vi "Main-Strech DNA-OneDirectionOnly_YCC.vi"() -> ()   [LabVIEW 2014]
uses:
  <vilib>/DAQmx/create/channels.llb/DAQmx Create Channel (AI-Voltage-Basic).vi
  <vilib>/DAQmx/configure/timing.llb/DAQmx Timing (Sample Clock).vi
  Main-Calibration/WLC fitting/SubVI/WLC-Fitting Cluster.ctl
panel:
  out "Fold QPD Signal (V) 2":dbl[](array[numeric])
  out "Fold Stage Position (um) 2":dbl[](array[numeric])
  out "Folded-Force":dbl[](array[numeric])
  out "Folded-xDNA":dbl[](array[numeric])
  out "Unfolded-Force":dbl[](array[numeric])
  out "Unfolded-xDNA":dbl[](array[numeric])
  in  "Fitting Cluster":T1={"cr (um)"=0.0, "yr (V)"=0.0, "trap height(nm)"=300.0, "bead radius(nm)"=515.0, "Length offset"=0.0, "conversion factor (V/um)"=0.0, "Force constant (pN/nm)"=0.0154, "Force offset"=500.0, "cr shift (nm)"=0.0, "yr shift (mV)"=0.0, "LaserPower (mW)"=10.0, "Cf. Calib. Array"=[0.192406, 0.0124489], "Stiffness Calib. array"=[0.004414, 0.00367]}
  out "Filtered QPD Array":dbl[][](array[numeric])
  out "Filtered Stage Array":dbl[][](array[numeric])
  out "Save to File Name Indicator":string
  out "Save to Path Indicator":path
  in  "Who's Data":enum16{"YCC", "PYW", "LCH"}(ring)
  in  "File name add to the end \n(laser power-height)":string="10mW-h300"
  in  "Save Raw Data?":bool
  out "Array 3":bool[](array[boolean])
  out "Array 2":dbl[](array[numeric])
  out "Array":dbl[](array[numeric])
  out "initial position offset after move":dbl[](array[numeric])
  out "Avg. to Hz":dbl
  out "Fold QPD Signal (V)":dbl[](array[numeric])
  out "Unfold QPD Signal (V)":dbl[](array[numeric])
  out "Fold Stage Position (um)":dbl[](array[numeric])
  out "Unfold Stage Position (um)":dbl[](array[numeric])
  in  "Tab Control":T2(tab)
  out "Stage-QPD Graph":T3(graph)
  out "Unfolded Graph":cluster{dbl[], dbl[]}(graph)
  out "Folded Graph":cluster{dbl[], dbl[]}(graph)
  out "Unfolded+Folded Graph":T4(graph)
  out "Stage-QPD Graph 2":T3(graph)
  in  "range  (um)":dbl=2.0 format="%.3f"
  in  "Record scan rate  (um/s)":dbl=2.0 format="%.3f"
  out "Trace direction":bool[](array[boolean])=[FALSE, TRUE, TRUE, FALSE]
  in  "Avg points":i32=200
  in  "Filter type":T5(ring)
  out "Real initial position (um)":dbl format="%0.5f"
  in  "Toward first ?\nT=+, F=-":bool
  in  "Record Mode \npath(1,2)":bool[](array[boolean])=[FALSE, FALSE, FALSE, FALSE]
  in  "Sampling rate":dbl=20000.0 format="%0.2f"
  in  "QPD value":dbl=1.0 format="%0.2f"
  in  "T=X\nF=Y":bool=TRUE
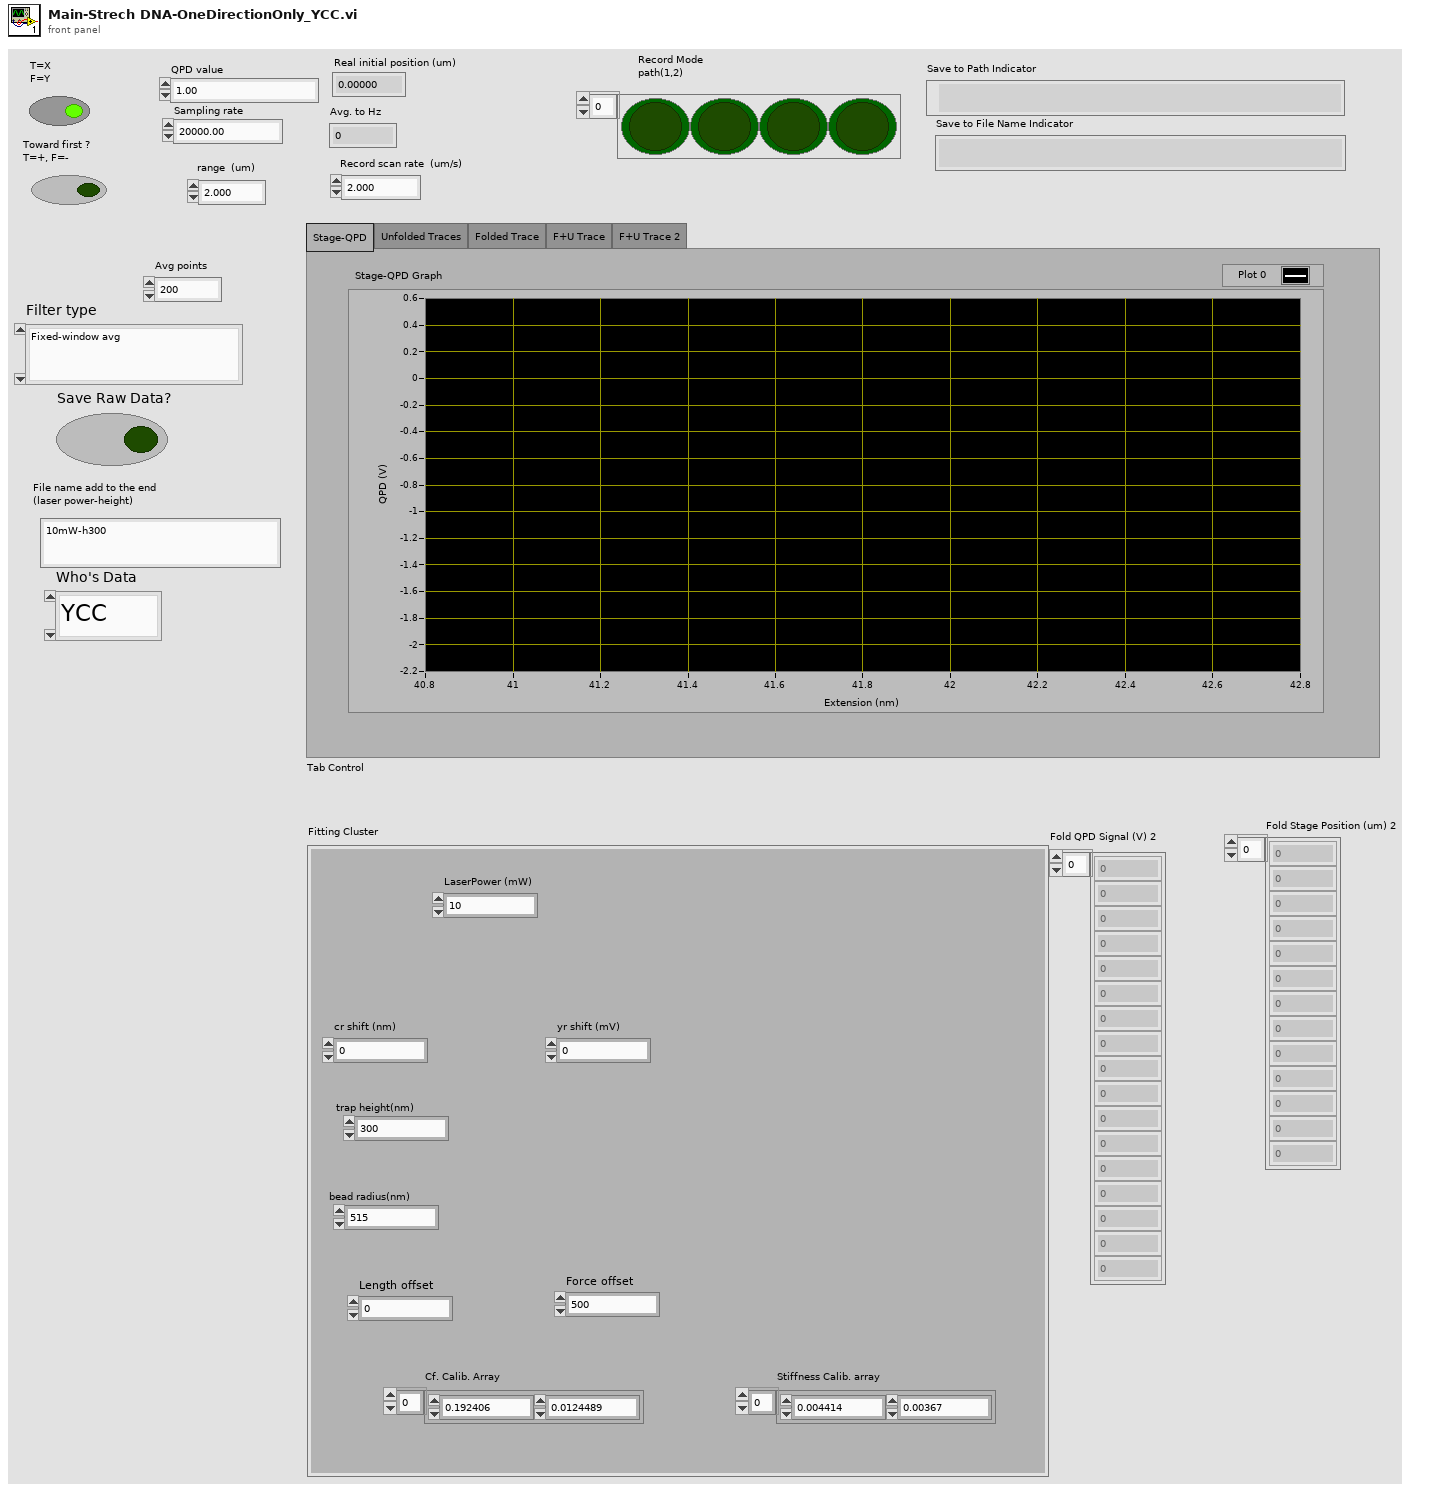
[diagram p1: front panel]
types:
  T1 = typedef "WLC-Fitting Cluster.ctl" = cluster{"cr (um)":dbl, "yr (V)":dbl, "trap height(nm)":dbl, "bead radius(nm)":dbl, "Length offset":dbl, "conversion factor (V/um)":dbl, "Force constant (pN/nm)":dbl, "Force offset":dbl, "cr shift (nm)":dbl, "yr shift (mV)":dbl, "LaserPower (mW)":dbl, "Cf. Calib. Array":dbl[], "Stiffness Calib. array":dbl[]}
  T2 = enum32{"Stage-QPD", "Unfolded Traces", "Folded Trace", "F+U Trace", "F+U Trace 2"}
  T3 = cluster{"Fold Stage Position (um)":dbl[], "Fold QPD Signal (V)":dbl[]}
  T4 = cluster{"Filtered Stage Array":dbl[], "Filtered QPD Array":dbl[]}[]
  T5 = enum16{"Fixed-window avg", "Moving-window avg", "S-G filter", "Median filter"}
  T6 = cluster{"Unfolded-xDNA":dbl[], "Unfolded-Force":dbl[]}
  T7 = cluster{"Folded-xDNA":dbl[], "Folded-Force":dbl[]}
  T8 = cluster{"Folded-xDNA":dbl[], "Folded-Force":dbl[]}[]
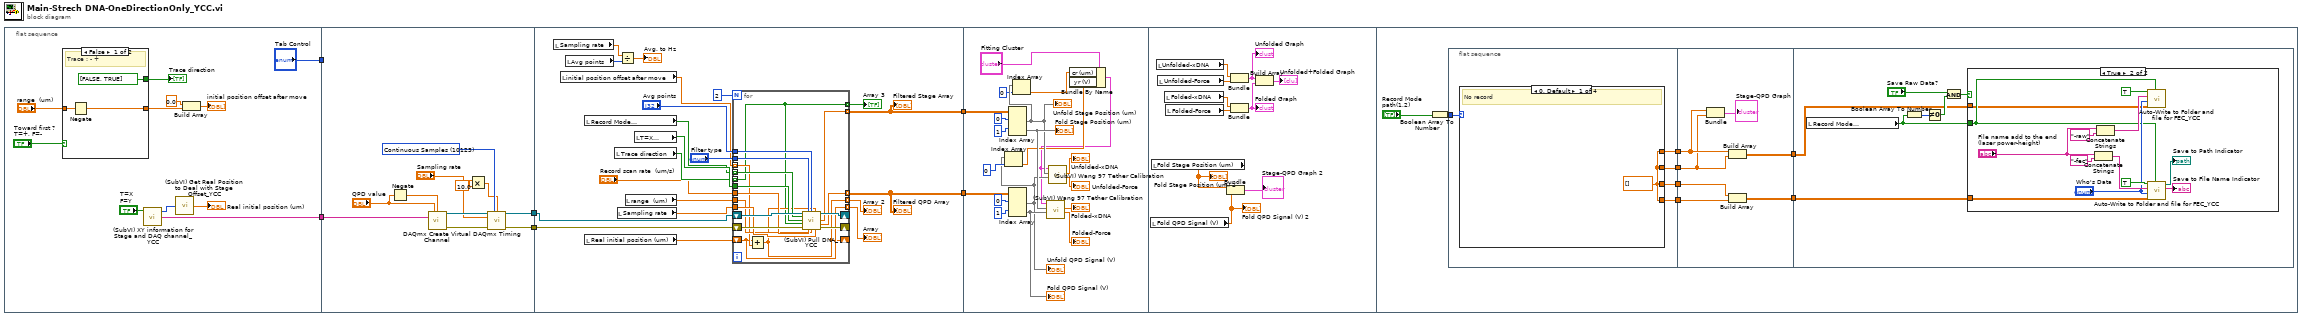
[diagram p0: block diagram]
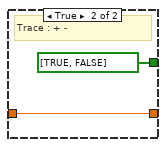
[diagram p2: hidden frame]
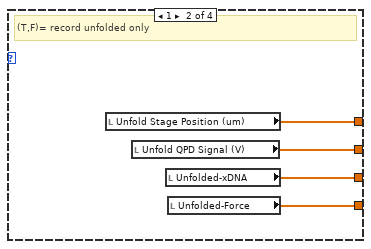
[diagram p3: hidden frame]
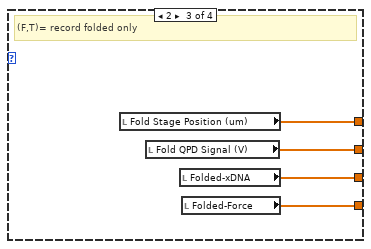
[diagram p4: hidden frame]
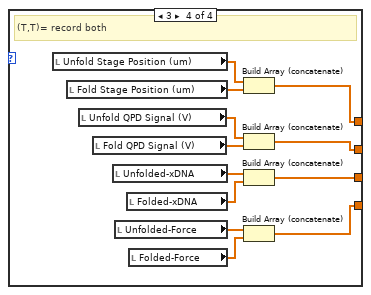
[diagram p5: hidden frame]
diagram:
  n1 = flat-sequence {
    tunnel: [w16] -> w6
    tunnel: ["Tab Control"] -> w3
    tunnel: w6 -> [w33]
    tunnel: [w27] -> w5
    tunnel: [w26] -> w4
    tunnel: w3 -> [_]
    tunnel: w5 -> [w38]
    tunnel: w4 -> [w37]
    tunnel: [w36] -> w2
    tunnel: [w35] -> w1
    tunnel: w1 -> [w86]
    tunnel: w2 -> [w91]
    frame #0 {
      n2 = case shown="False" "Toward first ?\nT=+, F=-" {
        tunnel: [bool[] [FALSE, TRUE] bool[] [TRUE, FALSE]] -> w12
        tunnel: "range  (um)" -> [w19 w21]
        tunnel: [w18 w21] -> w7
        frame False {
          # "Trace : - +"
          n3 = Negate(x=w19) -> (-x=w18:dbl)
        }
        frame True {
          # "Trace : + -"
        }
      }
      "Trace direction" <- w12
      n4 = call "(SubVI) XY information for Stage and DAQ channel_YCC.vi"("T=X\nF=Y"="T=X\nF=Y") -> ("physical channels"=w16:tag, "Axis"=w14:i32)  [unwired: 3 in]
      n5 = call "(SubVI) Get Real Position to Deal with Stage Offset_YCC.vi"("Axis"=w14) -> ("Real Current Commanded position (um)"=→"Real initial position (um)":dbl)  [unwired: 3 in, 1 out]
      n6 = Build Array(0.0, w7) -> (→"initial position offset after move":dbl[])
    }
    frame #1 {
      w28 = 10123 items=["Finite Samples"=10178, "Continuous Samples"=10123, "Hardware Timed Single Point"=12522] ("sample mode")
      n7 = Negate(x="QPD value") -> (-x=w29:dbl)
      n8 = call-poly <vilib>:"DAQmx Create Virtual Channel.vi"("maximum value"="QPD value", "minimum value"=w29, "physical channels"=w33) -> ("task out"=w31:refnum<k21>, "error out"=w32:errorcluster)  [unwired: 11 in]
      n9 = Multiply(x="Sampling rate", y=10.0) -> (x*y=w23:dbl)
      n10 = call-poly <vilib>:"DAQmx Timing.vi"("task/channels in"=w31, "sample mode"=w28, "samples per channel"=w23, "rate"="Sampling rate", "error in"=w32) -> ("task out"=w27:refnum<k21>, "error out"=w26:errorcluster)  [unwired: 9 in]
    }
    frame #2 {
      n11 = local read "Sampling rate"() -> (w46:dbl)
      n12 = local read "initial position offset after move"() -> (w42:dbl[])
      n13 = local read "Avg points"() -> (w45:i32)
      n14 = local read "Record Mode \npath(1,2)"() -> (w48:bool[])
      n15 = local read "Real initial position (um)"() -> (w50:dbl)
      n16 = local read "Trace direction"() -> (w51:bool[])
      n17 = local read "Sampling rate"() -> (w49:dbl)
      n18 = Divide(x=w46, y=w45) -> (x/y=→"Avg. to Hz":dbl)
      n19 = local read "range  (um)"() -> (w43:dbl)
      n20 = local read "T=X\nF=Y"() -> (w52:bool)
      n21 = for {
        N: 2 -> [_]
        shift-right: [w70] -> _
        shift-left: w38 -> [w71]
        shift-right: [w68] -> _
        shift-left: w37 -> [w69]
        tunnel: "Avg points" -> [w67]
        tunnel: "Filter type" -> [w66]
        tunnel: w48 -> [w65] mode=indexing
        tunnel: w52 -> [w64]
        tunnel: w51 -> [w55] mode=indexing
        tunnel: w49 -> [w63]
        tunnel: "Record scan rate  (um/s)" -> [w62]
        tunnel: w43 -> [w61]
        tunnel: [w60] -> w36 mode=indexing
        tunnel: [w59] -> w35 mode=indexing
        shift-right: [w56] -> _
        shift-left: w50 -> [w57]
        tunnel: w42 -> [w58] mode=indexing
        tunnel: [w57] -> w41 mode=indexing
        tunnel: [w56] -> w40 mode=indexing
        tunnel: [w55] -> w39 mode=indexing
        n22 = Add(x=w57, y=w58) -> (x+y=w56:dbl)
        n23 = call "(SubVI) Pull DNA_YCC.vi"("task/channels in"=w71, "Filter type"=w66, "Avg points"=w67, "Real initial position (um)"=w56, "Record?"=w65, "T=X\nF=Y"=w64, "Toward  ?\nT=+, F=-"=w55, "error in"=w69, "Record scan rate  (um/s)"=w62, "range  (um)"=w61, "Sampling rate"=w63) -> ("task out"=w70:refnum<k21>, "Filtered Stage Array"=w60:dbl[], "Filtered QPD Array"=w59:dbl[], "error out"=w68:errorcluster)  [unwired: 1 out]
      }
      "Array" <- w41
      "Array 2" <- w40
      "Array 3" <- w39
      "Filtered Stage Array" <- w36
      "Filtered QPD Array" <- w35
    }
    frame #3 {
      n24 = Index Array(array=w91, index (row) #1=0 ("index (row)"), index (row) #2=1 ("index (row)")) -> (element #1=w78:dbl[], element #2=w83:dbl[])  [unwired: 2 in]
      "Unfold Stage Position (um)" <- w78
      "Fold Stage Position (um)" <- w83
      n25 = Index Array(array=w86, index (row) #1=0 ("index (row)"), index (row) #2=1 ("index (row)")) -> (element #1=w74:dbl[], element #2=w82:dbl[])  [unwired: 2 in]
      "Unfold QPD Signal (V)" <- w74
      "Fold QPD Signal (V)" <- w82
      n26 = Index Array(array=w74, index=0) -> (element=w73:dbl)
      n27 = Index Array(array=w78, index=0) -> (element=w76:dbl)
      n28 = Bundle By Name(cluster="Fitting Cluster", "cr (um)"=w76, "yr (V)"=w73) -> (w72:T1)
      n29 = call "(SubVI) Wang 97 Tether Calibration.vi"("QPD signal"=w82, "Stage Position"=w83, "Fitting Cluster"=w72) -> ("Force"=→"Folded-Force":dbl[], "xDNA"=→"Folded-xDNA":dbl[])  [unwired: 2 in, 1 out]
      n30 = call "(SubVI) Wang 97 Tether Calibration.vi"("QPD signal"=w74, "Stage Position"=w78, "Fitting Cluster"=w72) -> ("Force"=→"Unfolded-Force":dbl[], "xDNA"=→"Unfolded-xDNA":dbl[])  [unwired: 2 in, 1 out]
    }
    frame #4 {
      n31 = local read "Fold QPD Signal (V)"() -> (w92:dbl[])
      "Fold QPD Signal (V) 2" <- w92
      n32 = local read "Fold Stage Position (um)"() -> (w93:dbl[])
      "Fold Stage Position (um) 2" <- w93
      n33 = local read "Unfolded-xDNA"() -> (w101:dbl[])
      n34 = local read "Unfolded-Force"() -> (w100:dbl[])
      n35 = local read "Folded-xDNA"() -> (w98:dbl[])
      n36 = local read "Folded-Force"() -> (w97:dbl[])
      n37 = Bundle("Fold Stage Position (um)"=w93, "Fold QPD Signal (V)"=w92) -> (→"Stage-QPD Graph 2":T3)  [unwired: 1 in]
      n38 = Bundle("Unfolded-xDNA"=w101, "Unfolded-Force"=w100) -> (w99:T6)  [unwired: 1 in]
      "Unfolded Graph" <- w99
      n39 = Bundle("Folded-xDNA"=w98, "Folded-Force"=w97) -> (w95:T7)  [unwired: 1 in]
      "Folded Graph" <- w95
      n40 = Build Array(w99, w95) -> (→"Unfolded+Folded Graph":T8)
    }
    frame #5 {
      n41 = Boolean Array To Number(Boolean array="Record Mode \npath(1,2)") -> (number=w108:u32)
      n42 = flat-sequence {
        tunnel: w108 -> [w112]
        tunnel: [w114] -> w107
        tunnel: [w113] -> w106
        tunnel: [w111] -> w104
        tunnel: [w110] -> w103
        tunnel: w107 -> [w138]
        tunnel: w106 -> [w137]
        tunnel: [w142] -> w105
        tunnel: w104 -> [w141]
        tunnel: w103 -> [w140]
        tunnel: [w139] -> w102
        tunnel: w105 -> [w146]
        tunnel: w102 -> [w143]
        frame #0 {
          n43 = case shown="0, Default" w112 {
            tunnel: [w115 w119 w123 w131] -> w114
            tunnel: [w115 w118 w122 w130] -> w113
            tunnel: [w115 w117 w121 w125] -> w111
            tunnel: [w115 w116 w120 w124] -> w110
            frame 0, Default {
              w115 = dbl[] [] ("Fold Stage Position (um)")
              # "No record"
            }
            frame 1 {
              # "(T,F)= record unfolded only"
              n44 = local read "Unfold Stage Position (um)"() -> (w119:dbl[])
              n45 = local read "Unfold QPD Signal (V)"() -> (w118:dbl[])
              n46 = local read "Unfolded-xDNA"() -> (w117:dbl[])
              n47 = local read "Unfolded-Force"() -> (w116:dbl[])
            }
            frame 2 {
              # "(F,T)= record folded only"
              n48 = local read "Fold Stage Position (um)"() -> (w123:dbl[])
              n49 = local read "Fold QPD Signal (V)"() -> (w122:dbl[])
              n50 = local read "Folded-xDNA"() -> (w121:dbl[])
              n51 = local read "Folded-Force"() -> (w120:dbl[])
            }
            frame 3 {
              # "(T,T)= record both"
              n52 = local read "Unfold Stage Position (um)"() -> (w135:dbl[])
              n53 = local read "Fold Stage Position (um)"() -> (w134:dbl[])
              n54 = local read "Unfold QPD Signal (V)"() -> (w133:dbl[])
              n55 = local read "Fold QPD Signal (V)"() -> (w132:dbl[])
              n56 = local read "Unfolded-xDNA"() -> (w129:dbl[])
              n57 = local read "Unfolded-Force"() -> (w127:dbl[])
              n58 = local read "Folded-xDNA"() -> (w128:dbl[])
              n59 = local read "Folded-Force"() -> (w126:dbl[])
              n60 = Build Array (concatenate)(w135, w134) -> (w131:dbl[])
              n61 = Build Array (concatenate)(w133, w132) -> (w130:dbl[])
              n62 = Build Array (concatenate)(w129, w128) -> (w125:dbl[])
              n63 = Build Array (concatenate)(w127, w126) -> (w124:dbl[])
            }
          }
        }
        frame #1 {
          n64 = Bundle("Fold Stage Position (um)"=w138, "Fold QPD Signal (V)"=w137) -> (→"Stage-QPD Graph":T3)  [unwired: 1 in]
          n65 = Build Array(w138, w137) -> (w142:dbl[][])
          n66 = Build Array(w141, w140) -> (w139:dbl[][])
        }
        frame #2 {
          n67 = local read "Record Mode \npath(1,2)"() -> (w144:bool[])
          n68 = Boolean Array To Number(Boolean array=w144) -> (number=w145:u32)
          n69 = Not Equal To 0?(x=w145) -> (x != 0?=w148:bool)
          n70 = And(x="Save Raw Data?", y=w148) -> (x .and. y?=w147:bool)
          n71 = case shown="True" w147 {
            tunnel: w146 -> [_ w150]
            tunnel: w144 -> [_ w152]
            tunnel: w143 -> [_ w151]
            frame False {
            }
            frame True {
              n72 = Concatenate Strings("File name add to the end \n(laser power-height)", "-fec" ("string")) -> (w157:string)
              n73 = Concatenate Strings("File name add to the end \n(laser power-height)", "-raw" ("string")) -> (w154:string)
              n74 = call "Auto-Write to Folder and file for FEC_YCC.vi"("Record Mode \npath(1,2)"=w152, "data to be saved"=w150, "Who's Data"="Who's Data", "File name add to the end \n(height)"=w154, "Save?"=TRUE) -> ()  [unwired: 3 in, 2 out]
              n75 = call "Auto-Write to Folder and file for FEC_YCC.vi"("Record Mode \npath(1,2)"=w152, "data to be saved"=w151, "Who's Data"="Who's Data", "File name add to the end \n(height)"=w157, "Save?"=TRUE) -> ("Save to File Name"=→"Save to File Name Indicator":string, "Save to Path"=→"Save to Path Indicator":path)  [unwired: 3 in]
            }
          }
        }
      }
    }
  }
